vi "server.vi"() -> ()   [LabVIEW 2020]
panel:
  in  "stop":bool
  in  "Tamper":cluster{u32, u32}[](array[cluster])
  in  "Bypass":cluster{u32, u32}[](array[cluster])
  in  "Alarm":cluster{u32, u32}[](array[cluster])
  in  "Normal":cluster{u32, u32}[](array[cluster])
  out "?":bool
  # "Green : Normal\nRed : Alarm\nBlue : Bypass\nOrange: Tamper"
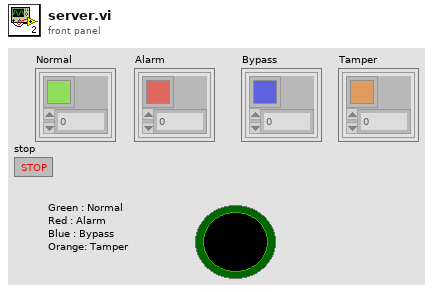
[diagram p1: front panel]
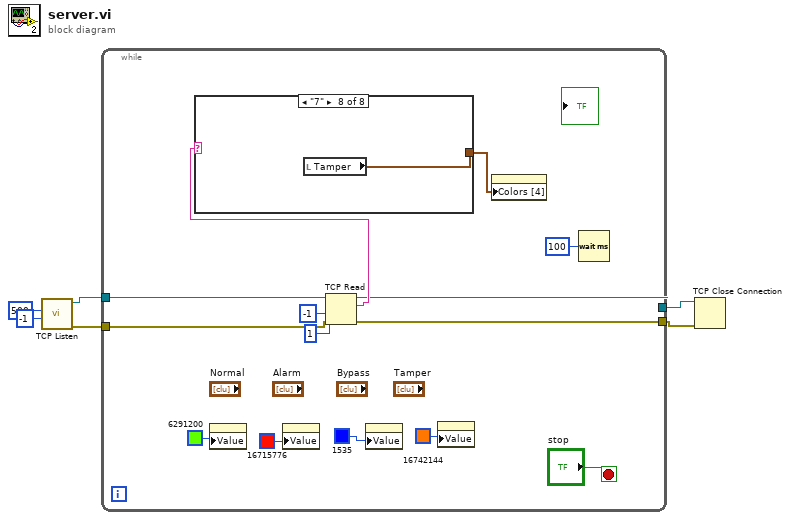
[diagram p0: block diagram]
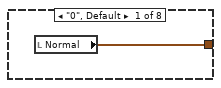
[diagram p2: hidden frame]
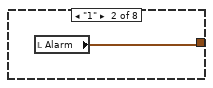
[diagram p3: hidden frame]
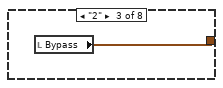
[diagram p4: hidden frame]
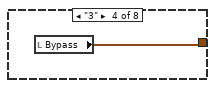
[diagram p5: hidden frame]
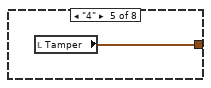
[diagram p6: hidden frame]
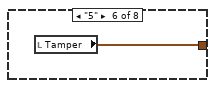
[diagram p7: hidden frame]
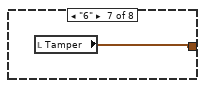
[diagram p8: hidden frame]
diagram:
  n1 = call <vilib>:"TCP Listen.vi"("timeout ms (wait forever: -1)"=-1, "port"=u16 500) -> ("error out"=w3:errorcluster, "connection ID"=w4:refnum<k5>)  [unwired: 5 in, 3 out]
  n2 = while {
    tunnel: w4 -> [w18]
    tunnel: w3 -> [w17]
    tunnel: [w16] -> w2
    tunnel: [w8] -> w1
    stop <- "stop" stop-if-true
    n3 = property class="ColBox"("Value"=u32 6291200) -> ()  [unwired: 2 in, 2 out]
    n4 = property class="ColBox"("Value"=u32 16715776) -> ()  [unwired: 2 in, 2 out]
    n5 = TCP Read(connection ID=w18, bytes to read=1, error in (no error)=w17, 9:-1 ("timeout ms (25000)")) -> (connection ID out=w8:refnum<k5>, data out=w15:string, error out=w16:errorcluster)  [unwired: 1 in]
    n6 = case shown="\"7\"" w15 {
      tunnel: [w21 w22 w23 w24 w25 w26 w27 w28] -> w14
      frame "0", Default {
        n7 = local read "Normal"() -> (w21:cluster{u32, u32}[])
      }
      frame "1" {
        n8 = local read "Alarm"() -> (w22:cluster{u32, u32}[])
      }
      frame "2" {
        n9 = local read "Bypass"() -> (w23:cluster{u32, u32}[])
      }
      frame "3" {
        n10 = local read "Bypass"() -> (w24:cluster{u32, u32}[])
      }
      frame "4" {
        n11 = local read "Tamper"() -> (w25:cluster{u32, u32}[])
      }
      frame "5" {
        n12 = local read "Tamper"() -> (w26:cluster{u32, u32}[])
      }
      frame "6" {
        n13 = local read "Tamper"() -> (w27:cluster{u32, u32}[])
      }
      frame "7" {
        n14 = local read "Tamper"() -> (w28:cluster{u32, u32}[])
      }
    }
    n15 = property class="ColBox"("Value"=u32 1535) -> ()  [unwired: 2 in, 2 out]
    n16 = property class="ColBox"("Value"=u32 16742144) -> ()  [unwired: 2 in, 2 out]
    n17 = property class="Bool (strict)"("Colors [4]"=w14) -> ()  [unwired: 2 in, 2 out]
    n18 = Wait (ms)(milliseconds to wait=u32 100) -> ()  [unwired: 1 out]
  }
  n19 = TCP Close Connection(connection ID=w1, error in (no error)=w2) -> ()  [unwired: 1 in, 2 out]
